vi "Merge Overlays.vi"(8 "error in (no error)":errorcluster, 11 "Overlay Filters":refnum<class "Overlay Filter.lvclass">[](array[class])) -> (0 "error out":errorcluster, 3 "Merged Overlay":refnum<class "Overlay Filter.lvclass">)   [LabVIEW 2020, in "CDM-Config.lvlib" / "Overlay Filter.lvclass"]
uses:
  Overlay Filter.lvclass
  Overlay Filter.lvclass/Overlay Filter.ctl
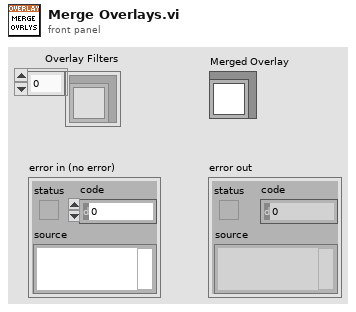
[diagram p1: front panel]
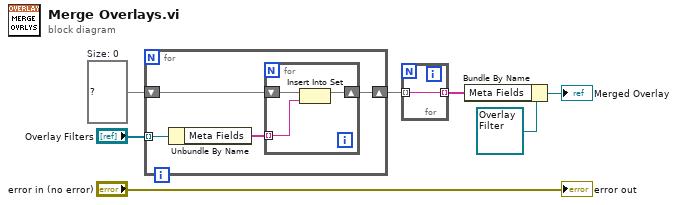
[diagram p0: block diagram]
diagram:
  w5 = set{string} {}  # Size: 0
  n1 = for {
    tunnel: "Overlay Filters" -> [w11] mode=indexing
    shift-right: [w8] -> w4
    shift-left: w5 -> [w10]
    n2 = Unbundle By Name(w11) -> ("Meta Fields"=w9:string[])
    n3 = for {
      tunnel: w9 -> [w13] mode=indexing
      shift-right: [w12] -> w8
      shift-left: w10 -> [w14]
      n4 = Insert Into Set(10:w13, 11:w14) -> (3:w12:set{string})  [unwired: 1 out]
    }
  }
  n5 = for {
    tunnel: w4 -> [w15] mode=indexing
    tunnel: [w15] -> w1 mode=indexing
  }
  n6 = Bundle By Name(cluster=refnum<class "Overlay Filter.lvclass"> refnum ("Merged Overlay"), "Meta Fields"=w1) -> (→"Merged Overlay":refnum<class "Overlay Filter.lvclass">)
  "error out" <- "error in (no error)"
